vi "identify and prepare loop timer source.vi"(8 "error in":errorcluster, 9 "module configs":refnum<class "TBM module configuration.lvclass">[](array[class]), 10 "module runtimes":refnum<class "TBM module execution interface.lvclass">[](array[class]), 11 "Standard Engine Configuration":refnum<class "Standard Engine Configuration.lvclass">) -> (0 "error out":errorcluster, 3 "timed loop timer source":T1={"Processor"=-2, "Priority"=0, "timing source dt"=5000, "timer source"=refnum})   [LabVIEW 2013, in "Standard Engine Runtime.lvclass"]
doc: "Identifies the timing source used for execution of the engine and prepares the inforation that it will need. This VI will also reserve CPU cores for execution if configured to do so."
uses:
  Standard Engine Runtime.lvclass
  <vilib>/NI/Tag Bus Module Framework/runtime/TBM module execution interface.lvclass
  Configuration/Standard Engine Configuration.lvclass
  <vilib>/NI/Tag Bus Module Framework/module configuration/TBM module configuration.lvclass
  main engine/timed loop timing sources.ctl
  <vilib>/NI/Module Timing Source/timing source/TBM timing source.lvclass
  Configuration/Standard Engine Configuration.lvclass/Standard Engine Configuration.ctl
  <vilib>/NI/Configuration Framework/serializable configuration/NISE_CEF_serializable configuration.lvclass/NISE_CEF_serializable configuration.ctl
  <vilib>/NI/Module Timing Source/standard timing source/ms timing source.lvclass
  <vilib>/NI/Module Timing Source/usec timing source/usec timing source.lvclass
  <vilib>/NI/Module Timing Source/scan engine timing source/scan engine timing source.lvclass
  Configuration/Read Processor.vi
  Configuration/Read Priority.vi
  Configuration/Read Master Timing Module.vi
  Configuration/Read Timing Source Type.vi
  Configuration/Read Timing Source dt.vi
  <vilib>/Utility/LVClass/Get LV Class Name.vi
  <vilib>/NI/Configuration Framework/error generator/NISE_error generator.vi
  <vilib>/NI/Configuration Framework/serializable configuration/NISE_CEF_serializable configuration.lvclass
  main engine/main engine.lvlib
  <vilib>/Utility/RT CPU pool selections.ctl
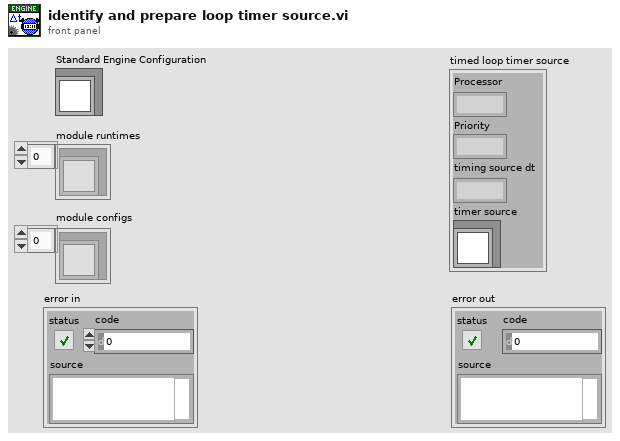
[diagram p1: front panel]
types:
  T1 = typedef "main engine.lvlib/timed loop timing sources.ctl" = cluster{"Processor":i32, "Priority":i32, "timing source dt":u32, "timer source":refnum<class "TBM timing source.lvclass">}
  T2 = typedef "Standard Engine Configuration.lvclass/Supported Timing Sources.ctl" = enum16{"Use Module Timing Source", "1 kHz Clock", "1 MHz Clock", "Synchronize to Scan Engine"}
  T3 = typedef "NI_Real-Time Target Support.lvlib/RT CPU pool selections.ctl" = enum16{"System & Timed Structures", "System", "Timed Structures", "Reserved"}
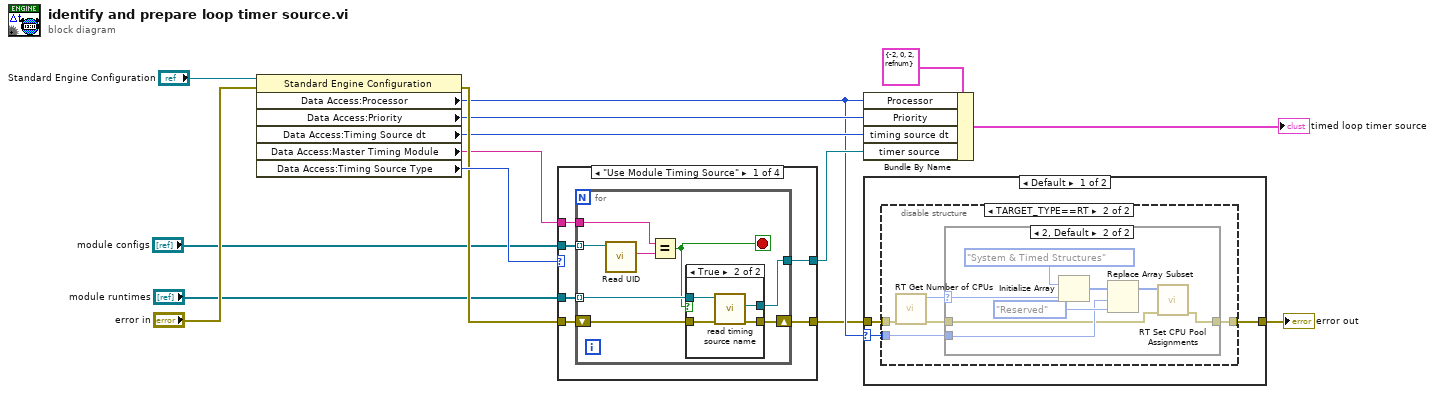
[diagram p0: block diagram]
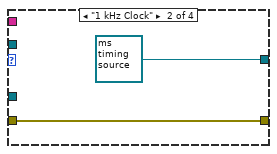
[diagram p6: hidden frame]
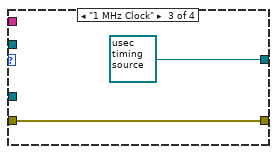
[diagram p7: hidden frame]
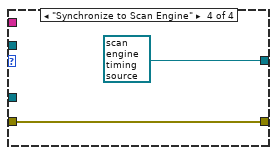
[diagram p8: hidden frame]
diagram:
  n1 = property class="Standard Engine Configuration"(reference="Standard Engine Configuration", error in="error in") -> (error out=w12:errorcluster, "Data Access:Processor"=w4:i32, "Data Access:Priority"=w7:i32, "Data Access:Timing Source dt"=w6:u32, "Data Access:Master Timing Module"=w9:string, "Data Access:Timing Source Type"=w13:T2)  [unwired: 1 out]
  n2 = case shown="\"Use Module Timing Source\"" w13 {
    tunnel: [w19 refnum<class "ms timing source.lvclass"> refnum ("ms timing source.lvclass") refnum<class "usec timing source.lvclass"> refnum ("usec timing source.lvclass") refnum<class "scan engine timing source.lvclass"> refnum ("scan engine timing source.lvclass")] -> w5
    tunnel: "module configs" -> [w21 _ _ _]
    tunnel: "module runtimes" -> [w20 _ _ _]
    tunnel: [w18 w35 w37 w39] -> w3
    tunnel: w12 -> [w17 w35 w37 w39]
    tunnel: w9 -> [w16 _ _ _]
    frame "Use Module Timing Source" {
      n3 = for {
        tunnel: w21 -> [w29] mode=indexing
        tunnel: w20 -> [w27] mode=indexing
        tunnel: [w25] -> w19
        shift-right: [w24] -> w18
        shift-left: w17 -> [w23]
        tunnel: w16 -> [w22]
        stop <- w26 stop-if-true
        n4 = call <vilib>:"Read UID.vi"("configuration in"=w29) -> ("instance id"=w28:string)  [unwired: 8 in, 2 out]
        n5 = Equal?(x=w22, y=w28) -> (x = y?=w26:bool)
        n6 = case shown="True" w26 {
          tunnel: w27 -> [_ w34]
          tunnel: [_ w33] -> w25
          tunnel: [w30 w32] -> w24
          tunnel: w23 -> [w30 w31]
          frame False {
          }
          frame True {
            n7 = call-dynamic "read timing source name.vi"("error in"=w31, "module in"=w34) -> ("error out"=w32:errorcluster, "timing source"=w33:refnum<class "TBM timing source.lvclass">)  [unwired: 7 in, 1 out]
          }
        }
      }
    }
    frame "1 kHz Clock" {
    }
    frame "1 MHz Clock" {
    }
    frame "Synchronize to Scan Engine" {
    }
  }
  n8 = Bundle By Name(cluster=T1 {"Processor"=-2, "Priority"=0, "timing source dt"=2, "timer source"=refnum} ("timed loop timer source"), "Processor"=w4, "Priority"=w7, "timing source dt"=w6, "timer source"=w5) -> (→"timed loop timer source":T1)
  n9 = case shown="Default" w4 {
    selector: w4 -> [w41 _]
    tunnel: w3 -> [w43 w59]
    tunnel: [w42 w59] -> w2
    frame Default {
      n10 = disable-structure shown="TARGET_TYPE==RT" {
        disable-tunnel: w43 -> [w44 w48]
        disable-tunnel: w41 -> [_ w46]
        disable-tunnel: [w44 w45] -> w42
        frame condition #0 (active) {
        }
        frame condition #1 {
          n11 = call <vilib>:"RT Get Number of CPUs.vi"("error in (no error)"=w48) -> ("error out"=w47:errorcluster, "# of CPUs"=w49:u32)  [unwired: 9 in]
          n12 = case shown="2, Default" w49 {
            selector: w49 -> [_ w57]
            tunnel: w47 -> [w50 w52]
            tunnel: w46 -> [_ w54]
            tunnel: [w50 w51] -> w45
            frame 0, 1 {
            }
            frame 2, Default {
              n13 = Initialize Array(RT_CPU_pool_selections."System & Timed Structures" ("Enum"), w57) -> (w56:T3[])
              n14 = Replace Array Subset(array=w56, new element=RT_CPU_pool_selections."Reserved" ("new element/subarray"), index=w54) -> (w53:T3[])
              n15 = call <vilib>:"RT Set CPU Pool Assignments.vi"("error in (no error)"=w52, "CPU pools"=w53) -> ("error out"=w51:errorcluster)  [unwired: 6 in, 3 out]
            }
          }
        }
      }
    }
    frame -2 {
    }
  }
  "error out" <- w2
